vi "Read Test Label.vi"(8 "error in":errorcluster, 11 "Naming Data in":refnum<class "Naming Data.lvclass">) -> (0 "error out":errorcluster, 2 "Test Label":string, 3 "Naming Data out":refnum<class "Naming Data.lvclass">)   [LabVIEW 2020, in "Approval Tests.lvlib" / "Naming Data.lvclass"]
uses:
  Naming Data.lvclass
  Naming Data.lvclass/Naming Data.ctl
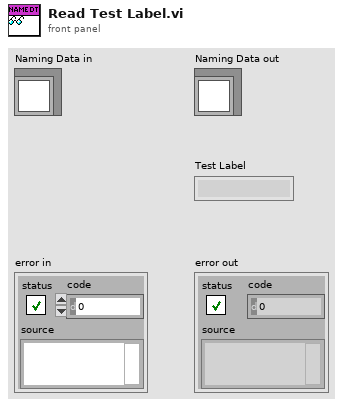
[diagram p1: front panel]
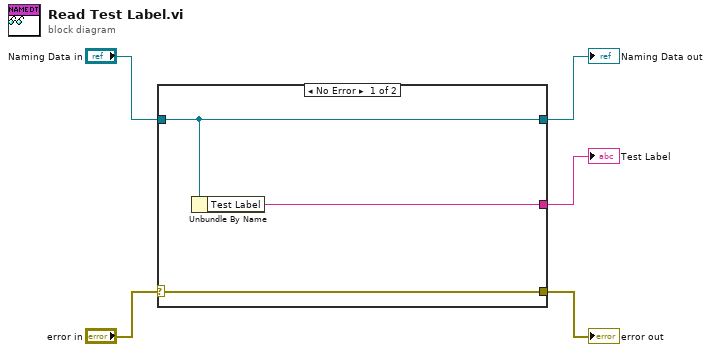
[diagram p0: block diagram]
diagram:
  n1 = case shown="No Error" "error in" {
    selector: "error in" -> [w8 w10]
    tunnel: [w8 w10] -> w4
    tunnel: [w7 w9] -> w2
    tunnel: "Naming Data in" -> [w7 w9]
    tunnel: [w6 _] -> w1
    frame No Error {
      n2 = Unbundle By Name(w7) -> ("Test Label"=w6:string)
    }
    frame Error {
    }
  }
  "error out" <- w4
  "Naming Data out" <- w2
  "Test Label" <- w1
